vi "Tile Same Size Pictures by Row and Col.vi"(6 "Rows and Cols":i32[](array[numeric]), 7 "Start Point":cluster{"x":i16, "y":i16} caption="Start (x,y)", 8 "错误输入":errorcluster, 9 "Para":T2={"Frame?"=FALSE, "Pen and Color"={"pen"={"Width"=1, "Style"=enum."Solid"}, "color(black)"=0}}, 10 "ImageData Array":T1[](array[typedef]), 11 "Picture in":picture) -> (0 "错误输出":errorcluster, 3 "Picture out":picture)   [LabVIEW 2012, in "Picture Box Tools.lvlib"]
uses:
  Picture Box Tools.lvlib
  <vilib>/picture/picture.llb/imagedata.ctl
  Rectangle Tools/Rect/OffsetRect/OffsetRect by Point and Rect.vi
  Rectangle Tools/Rect/Rect Tools.lvlib
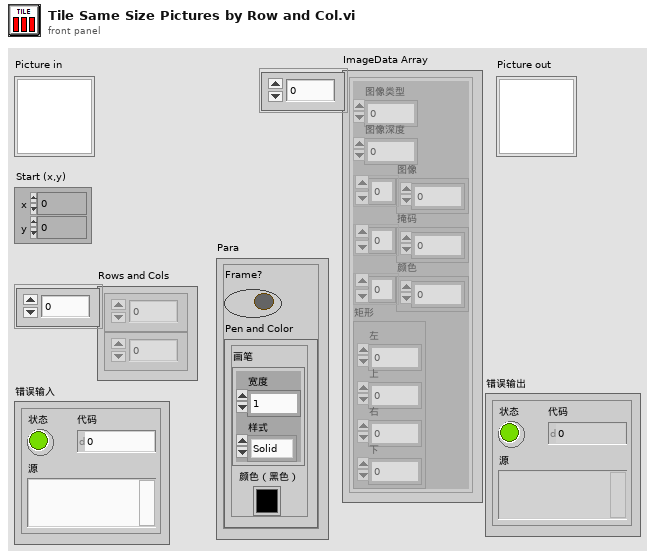
[diagram p1: front panel]
types:
  T1 = typedef "imagedata.ctl" = cluster{"image type":i32, "image depth":i32, "image":u8[], "mask":u8[], "colors":u32[], "Rectangle":cluster{"left":i16, "top":i16, "right":i16, "bottom":i16}}
  T2 = cluster{"Frame?":bool, "Pen and Color":cluster{"pen":cluster{"Width":i16, "Style":enum32{"Solid", "Dash", "Dot", "DashDot", "DashDotDot"}}, "color(black)":u32}}
  T3 = cluster{"pen":cluster{"Width":i16, "Style":enum32{"Solid", "Dash", "Dot", "DashDot", "DashDotDot"}}, "color(black)":u32}
  T4 = cluster{"left":i16, "top":i16, "right":i16, "bottom":i16}
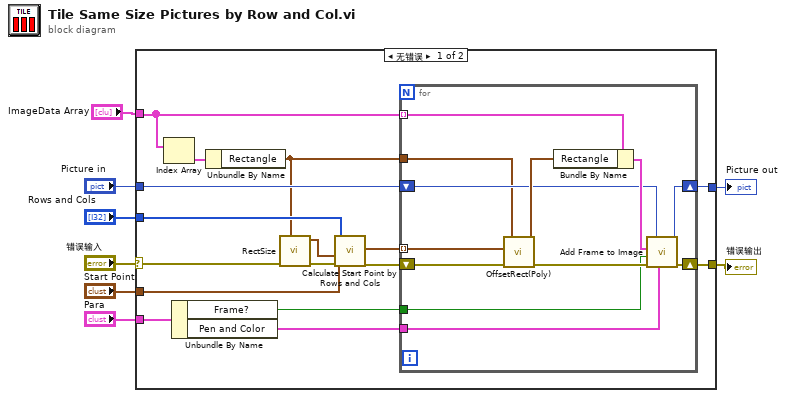
[diagram p0: block diagram]
diagram:
  n1 = case shown="无错误" "错误输入" {
    selector: "错误输入" -> [w14 w38]
    tunnel: [w17 w38] -> w7
    tunnel: "Picture in" -> [w16 w37]
    tunnel: [w18 w37] -> w5
    tunnel: "Para" -> [w24 _]
    tunnel: "Rows and Cols" -> [w23 _]
    tunnel: "Start Point" -> [w22 _]
    tunnel: "ImageData Array" -> [w11 _]
    frame No Error {
      n2 = Index Array(array=w11) -> (element=w10:T1)  [unwired: 1 in]
      n3 = Unbundle By Name(w24) -> ("Frame?"=w15:bool, "Pen and Color"=w19:T3)
      n4 = Unbundle By Name(w10) -> ("Rectangle"=w12:T4)
      n5 = call "RectSize.vi"("错误输入"=w14, "rect"=w12) -> ("错误输出"=w13:errorcluster, "point"=w9:cluster{"x":i16, "y":i16})  [unwired: 6 in, 2 out]
      n6 = call "Calculate Start Point by Rows and Cols.vi"("错误输入"=w13, "Size"=w9, "Start Point"=w22, "Rows and Cols"=w23) -> ("错误输出"=w20:errorcluster, "Start Point Array"=w21:cluster{"x":i16, "y":i16}[])  [unwired: 6 in]
      n7 = for {
        tunnel: w21 -> [w36] mode=indexing
        shift-right: [w29] -> w17
        shift-left: w20 -> [w35]
        shift-right: [w28] -> w18
        shift-left: w16 -> [w31]
        tunnel: w19 -> [w27]
        tunnel: w15 -> [w26]
        tunnel: w11 -> [w34] mode=indexing
        tunnel: w12 -> [w25]
        n8 = call-poly "OffsetRect(Poly).vi"("错误输入"=w35, "point"=w36, "rect"=w25) -> ("错误输出"=w30:errorcluster, "offset rect"=w33:T4)  [unwired: 7 in]
        n9 = Bundle By Name(cluster=w34, "Rectangle"=w33) -> (w32:T1)
        n10 = call "Add Frame to Image.vi"("Option"=w27, "错误输入"=w30, "Frame?"=w26, "image data"=w32, "Picture in"=w31) -> ("错误输出"=w29:errorcluster, "Picture out"=w28:picture)  [unwired: 5 in]
      }
    }
    frame Error {
    }
  }
  "Picture out" <- w5
  "错误输出" <- w7
